vi "Probability - Read.vi"(7 "QuWire in":refnum<class "QuWire.lvclass">) -> (8 "Probability":dbl[](array[numeric]))   [LabVIEW 2020]
uses:
  QuSim/QuWire/QuWire.lvclass
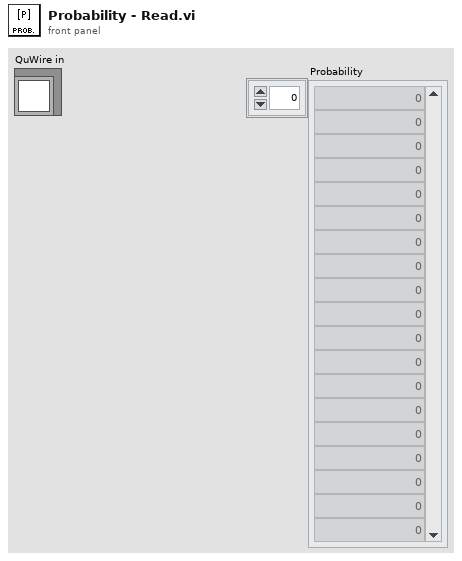
[diagram p1: front panel]
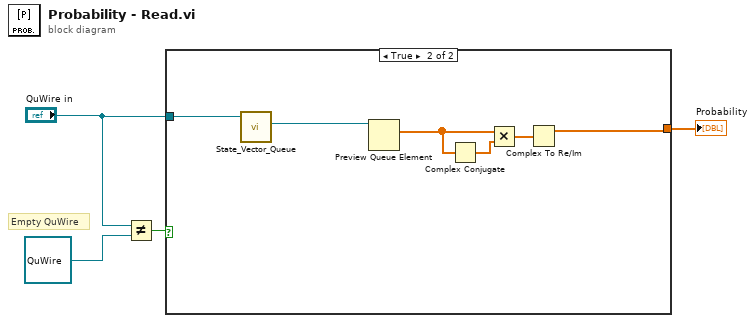
[diagram p0: block diagram]
diagram:
  # "Empty QuWire"
  n1 = Not Equal?(x="QuWire in", y=refnum<class "QuWire.lvclass"> refnum ("QuWire in")) -> (x != y?=w3:bool)
  n2 = case shown="True" w3 {
    tunnel: "QuWire in" -> [_ w5]
    tunnel: [_ w6] -> w1
    frame False {
    }
    frame True {
      n3 = call "State_Vector_Queue.vi"("QuWire in"=w5) -> ("State Vector Queue"=w10:refnum<queue>)  [unwired: 8 in, 2 out]
      n4 = Preview Queue Element(queue=w10) -> (element=w8:cdb[])  [unwired: 2 in, 3 out]
      n5 = Complex Conjugate(1:w8) -> (0:w9:cdb[])
      n6 = Multiply(x=w8, y=w9) -> (x*y=w7:cdb[])
      n7 = Complex To Re/Im(x + iy=w7) -> (x=w6:dbl[])  [unwired: 1 out]
    }
  }
  "Probability" <- w1
